vi "test_MonoMoveToPosition.vi"(0 "device selection":enum16{"monochromator", "CCD", "SCD"}(ring), 1 "Test should pass":bool=TRUE, 5 "set-up a connection":bool=TRUE, 9 "tear down connection":bool=TRUE, 11 "error in":errorcluster, 12 "Delay between send and receive [ms]":i32=100) -> (4 "first loop":i32, 6 "first loop 2":i32, 8 "first loop 3":i32, 10 "log-file path":path, 15 "error out":errorcluster)   [LabVIEW 2023]
uses:
  Classes/Mono/Monochromator.lvclass
  <vilib>/addons/_JKI Toolkits/Caraya/classes/Assert/Assert Not Error.vi
  <vilib>/addons/_JKI Toolkits/Caraya/classes/Test/Test.lvclass
  <vilib>/addons/_JKI Toolkits/Caraya/classes/Assert/Assert.lvclass
  <vilib>/Hampel Software Engineering/HSE Logger/hse-logger.lvlib
panel:
  # "Connector Pane"
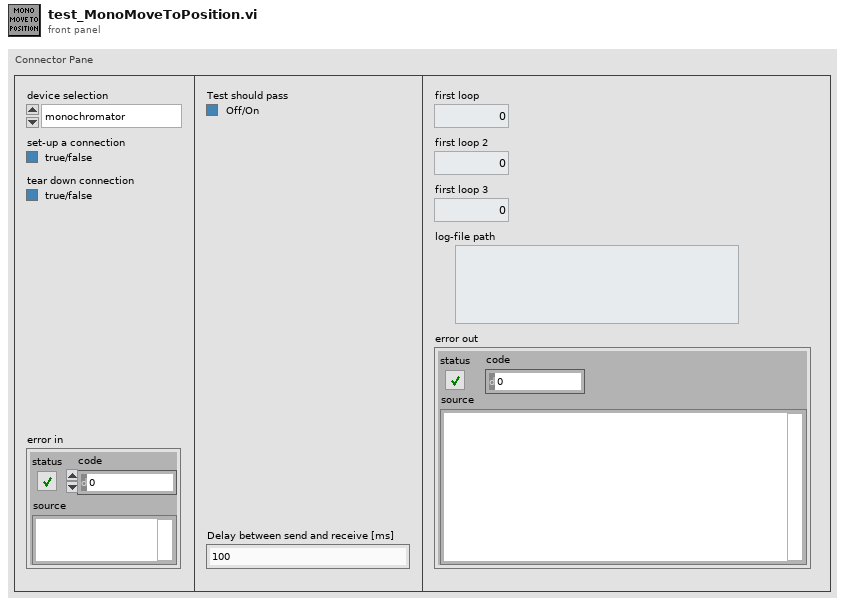
[diagram p1: front panel]
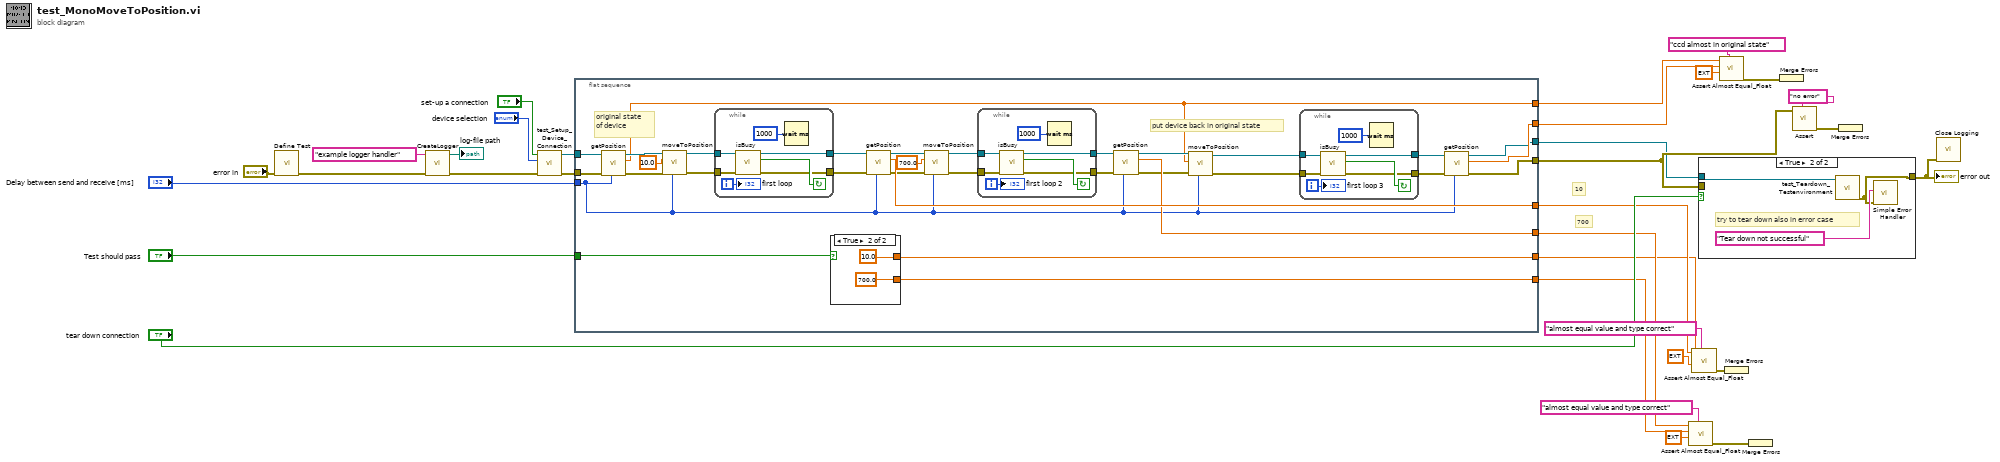
[diagram p0: block diagram]
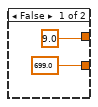
[diagram p2: hidden frame]
diagram:
  # "700"
  # "10"
  n1 = call <vilib>:"Define Test.vi"("error in (no error)"="error in") -> ("error out"=w11:errorcluster)  [unwired: 9 in, 1 out]
  n2 = call "CreateLogger.vi"("error in (no error)"=w11, "Handler Name"="example logger handler") -> ("error out"=w10:errorcluster, "log-file path"=→"log-file path":path)  [unwired: 8 in]
  n3 = call "test_Setup_Device_Connection.vi"("error in (no error)"=w10, "device selection"="device selection", "set-up a connection"="set-up a connection") -> ("error out"=w16:errorcluster, "Monochromator.lvclass"=w14:refnum<class "Monochromator.lvclass">)  [unwired: 5 in, 2 out]
  n4 = flat-sequence {
    tunnel: w16 -> [w60]
    tunnel: w14 -> [w61]
    tunnel: [w47] -> w26
    tunnel: "Test should pass" -> [w64]
    tunnel: [w48] -> w25
    tunnel: [w52] -> w24
    tunnel: [w63] -> w23
    tunnel: [w56] -> w7
    tunnel: [w62] -> w6
    tunnel: [w33] -> w20
    tunnel: [w49] -> w19
    tunnel: "Delay between send and receive [ms]" -> [w34]
    frame #0 {
      # "put device back in original state"
      # "original state of device"
      n5 = call "getPosition.vi"("Delay between send and receive [ms]"=w34, "error in (no error)"=w60, "Monochromator in"=w61) -> ("error out"=w58:errorcluster, "wavelength"=w33:dbl, "Monochromator out"=w59:refnum<class "Monochromator.lvclass">)  [unwired: 6 in]
      n6 = call "moveToPosition.vi"("Delay between send and receive [ms]"=w34, "error in (no error)"=w58, "wavelength"=10.0 ("exposure time [ms]"), "Monochromator in"=w59) -> ("error out"=w44:errorcluster, "Monochromator out"=w46:refnum<class "Monochromator.lvclass">)  [unwired: 4 in, 2 out]
      n7 = while {
        tunnel: w46 -> [w83]
        tunnel: [w82] -> w45
        tunnel: w44 -> [w81]
        tunnel: [w80] -> w43
        i -> [w79]
        stop <- w85 continue-if-true
        n8 = call "isBusy.vi"("error in (no error)"=w81, "Monochromator in"=w83) -> ("error out"=w80:errorcluster, "Mono is busy?"=w85:bool, "Monochromator out"=w82:refnum<class "Monochromator.lvclass">)  [unwired: 7 in]
        n9 = Wait (ms)(milliseconds to wait=u32 1000) -> ()  [unwired: 1 out]
        "first loop" <- w79
      }
      n10 = case shown="True" w64 {
        tunnel: [699.0 ("exposure time [ms]") 700.0 ("exposure time [ms]")] -> w63
        tunnel: [9.0 ("exposure time [ms]") 10.0 ("exposure time [ms]")] -> w62
        frame False {
        }
        frame True {
        }
      }
      n11 = call "getPosition.vi"("Delay between send and receive [ms]"=w34, "error in (no error)"=w43, "Monochromator in"=w45) -> ("error out"=w54:errorcluster, "wavelength"=w56:dbl, "Monochromator out"=w55:refnum<class "Monochromator.lvclass">)  [unwired: 6 in]
      n12 = call "moveToPosition.vi"("Delay between send and receive [ms]"=w34, "error in (no error)"=w54, "wavelength"=700.0 ("exposure time [ms]"), "Monochromator in"=w55) -> ("error out"=w41:errorcluster, "Monochromator out"=w42:refnum<class "Monochromator.lvclass">)  [unwired: 4 in, 2 out]
      n13 = while {
        tunnel: w42 -> [w76]
        tunnel: [w72] -> w39
        tunnel: w41 -> [w75]
        tunnel: [w74] -> w40
        i -> [w73]
        stop <- w78 continue-if-true
        n14 = call "isBusy.vi"("error in (no error)"=w75, "Monochromator in"=w76) -> ("error out"=w74:errorcluster, "Mono is busy?"=w78:bool, "Monochromator out"=w72:refnum<class "Monochromator.lvclass">)  [unwired: 7 in]
        n15 = Wait (ms)(milliseconds to wait=u32 1000) -> ()  [unwired: 1 out]
        "first loop 2" <- w73
      }
      n16 = call "getPosition.vi"("Delay between send and receive [ms]"=w34, "error in (no error)"=w40, "Monochromator in"=w39) -> ("error out"=w50:errorcluster, "wavelength"=w52:dbl, "Monochromator out"=w51:refnum<class "Monochromator.lvclass">)  [unwired: 6 in]
      n17 = call "moveToPosition.vi"("Delay between send and receive [ms]"=w34, "error in (no error)"=w50, "wavelength"=w33, "Monochromator in"=w51) -> ("error out"=w36:errorcluster, "Monochromator out"=w38:refnum<class "Monochromator.lvclass">)  [unwired: 4 in, 2 out]
      n18 = while {
        tunnel: w38 -> [w69]
        tunnel: [w65] -> w37
        tunnel: w36 -> [w68]
        tunnel: [w67] -> w35
        i -> [w66]
        stop <- w71 continue-if-true
        n19 = call "isBusy.vi"("error in (no error)"=w68, "Monochromator in"=w69) -> ("error out"=w67:errorcluster, "Mono is busy?"=w71:bool, "Monochromator out"=w65:refnum<class "Monochromator.lvclass">)  [unwired: 7 in]
        n20 = Wait (ms)(milliseconds to wait=u32 1000) -> ()  [unwired: 1 out]
        "first loop 3" <- w66
      }
      n21 = call "getPosition.vi"("Delay between send and receive [ms]"=w34, "error in (no error)"=w35, "Monochromator in"=w37) -> ("error out"=w47:errorcluster, "wavelength"=w49:dbl, "Monochromator out"=w48:refnum<class "Monochromator.lvclass">)  [unwired: 6 in]
    }
  }
  n22 = call <vilib>:"Assert Almost Equal_Float.vi"("Label"="almost equal value and type correct" ("Label (VI Title)"), "Tolerance"=ext 0.1, "Y"=w23, "X"=w24) -> ("error out"=w32:errorcluster)  [unwired: 6 in, 1 out]
  n23 = call <vilib>:"Assert Almost Equal_Float.vi"("Label"="almost equal value and type correct" ("Label (VI Title)"), "Tolerance"=ext 0.1, "Y"=w6, "X"=w7) -> ("error out"=w4:errorcluster)  [unwired: 6 in, 1 out]
  n24 = case shown="True" "tear down connection" {
    tunnel: w25 -> [_ w92]
    tunnel: [w90 w91] -> w9
    tunnel: w26 -> [w90 _]
    frame False {
    }
    frame True {
      # "try to tear down also in error case"
      n25 = call "test_Teardown_Testenvironment.vi"("GenericDevice.lvclass"=w92) -> ("error out"=w91:errorcluster)  [unwired: 9 in, 1 out]
      n26 = call <vilib>:"Simple Error Handler.vi"("error source (\" \")"="Tear down not successful" ("error source (\" \")"), "error in (no error)"=w91) -> ()  [unwired: 3 in, 5 out]
    }
  }
  "error out" <- w9
  n27 = call <vilib>:"Assert Almost Equal_Float.vi"("Label"="ccd almost in original state" ("Label (VI Title)"), "Tolerance"=ext 0.1, "Y"=w19, "X"=w20) -> ("error out"=w22:errorcluster)  [unwired: 6 in, 1 out]
  n28 = Merge Errors(w4) -> ()  [unwired: 1 out]
  n29 = Merge Errors(w32) -> ()  [unwired: 1 out]
  n30 = Merge Errors(w22) -> ()  [unwired: 1 out]
  n31 = call-poly <vilib>:"Assert.vi"("Label"="no error" ("Label (VI Title)"), "Not Error?"=w26) -> ("error out"=w28:errorcluster)  [unwired: 8 in, 1 out]
  n32 = Merge Errors(w28) -> ()  [unwired: 1 out]
  n33 = call <vilib>:"Close Logging.vi"("error in"=w9) -> ()  [unwired: 10 in, 1 out]
